vi "Report Local Error.vi"(8 "error in (no error)":errorcluster, 9 "Name":string, 10 "Path":path, 11 "VolatusAPI":refnum<class "VolatusAPI.lvclass">) -> ()   [LabVIEW 2020, in "VolatusSeqGUI.lvlib" / "Sequencing Control.lvclass"]
uses:
  Sequencing Control.lvclass
  Sequencing Control.lvclass/Sequencing Control.ctl
  Volatus/VolatusAPI/VolatusAPI.lvclass
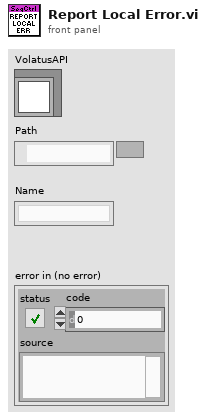
[diagram p1: front panel]
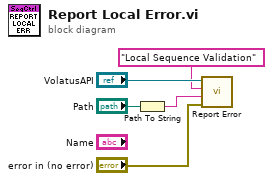
[diagram p0: block diagram]
diagram:
  n1 = Path To String(path="Path") -> (string=w2:string)
  n2 = call "Report Error.vi"("error in (no error)"="error in (no error)", "Message"=w2, "Context"="Local Sequence Validation", "VolatusAPI in"="VolatusAPI") -> ()  [unwired: 6 in, 2 out]
